vi "PAM Set Time TCP.vi"(7 "Error In":errorcluster {"code" format="%.0x"}, 10 "ID In":refnum<k5>) -> (0 "Error Out":errorcluster, 2 "Response":string, 3 "ID Out":refnum<k5>)   [LabVIEW 2020]
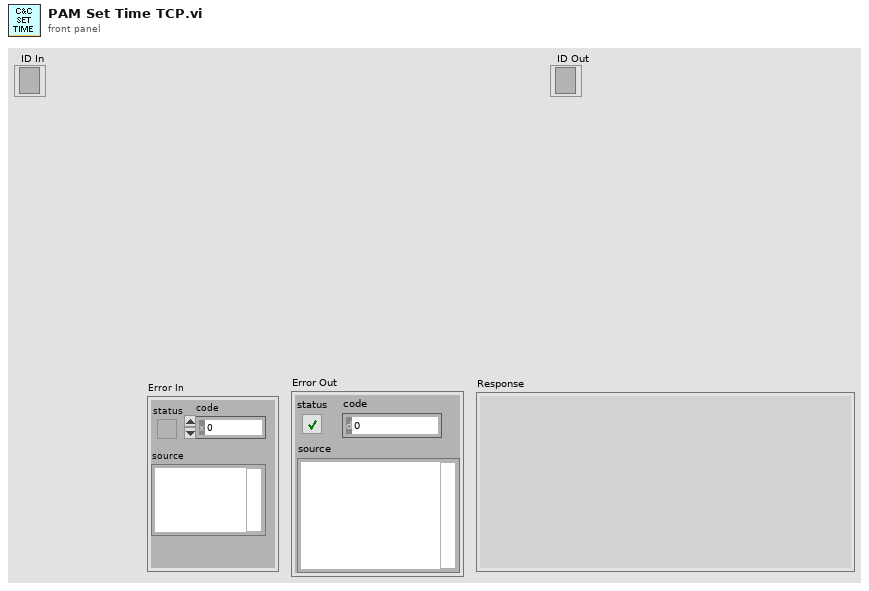
[diagram p1: front panel]
types:
  T1 = enum16{"big-endian, network order", "native, host order", "little-endian"}
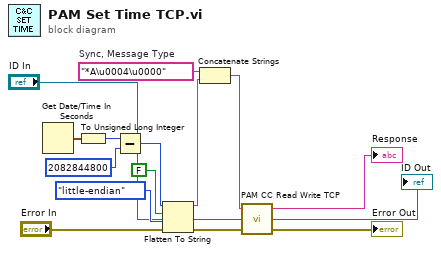
[diagram p0: block diagram]
diagram:
  w13 = "*A\u0004\u0000"  # Sync, Message Type
  n1 = Get Date/Time In Seconds() -> (seconds since 1Jan1904=w10:timestamp)
  n2 = To Unsigned Long Integer(number=w10) -> (unsigned 32bit integer=w11:u32)
  n3 = Subtract(x=w11, y=u32 2082844800) -> (x-y=w8:u32)
  n4 = Flatten To String(anything=w8, prepend array or string size? (T)=FALSE, byte order (0:big-endian, network order)=T1."little-endian", error in (no error)="Error In") -> (data string=w4:string, error out=w5:errorcluster)  [unwired: 1 out]
  n5 = Concatenate Strings(w13, w4) -> (w9:string)
  n6 = call "PAM CC Read Write TCP.vi"("Error In"=w5, "ID In"="ID In", "Command"=w9) -> ("Error Out"=→"Error Out":errorcluster, "ID Out"=→"ID Out":refnum<k5>, "Response"=→"Response":string)
